vi "名称未設定 1.vi"() -> ()   [LabVIEW 2016]
panel:
  in  "FieldPoint I/Oポイント":refnum<k21>
  in  "DAQmxデバイス名":tag
  in  "クラシック従来型DAQチャンネル":tag
  in  "クラシックDAQmxデバイス名":tag
  out "波形チャート 4":dbl(graph)
  out "波形チャート 3":dbl(graph)
  out "波形チャート 2":dbl(graph)
  out "波形チャート":dbl(graph)
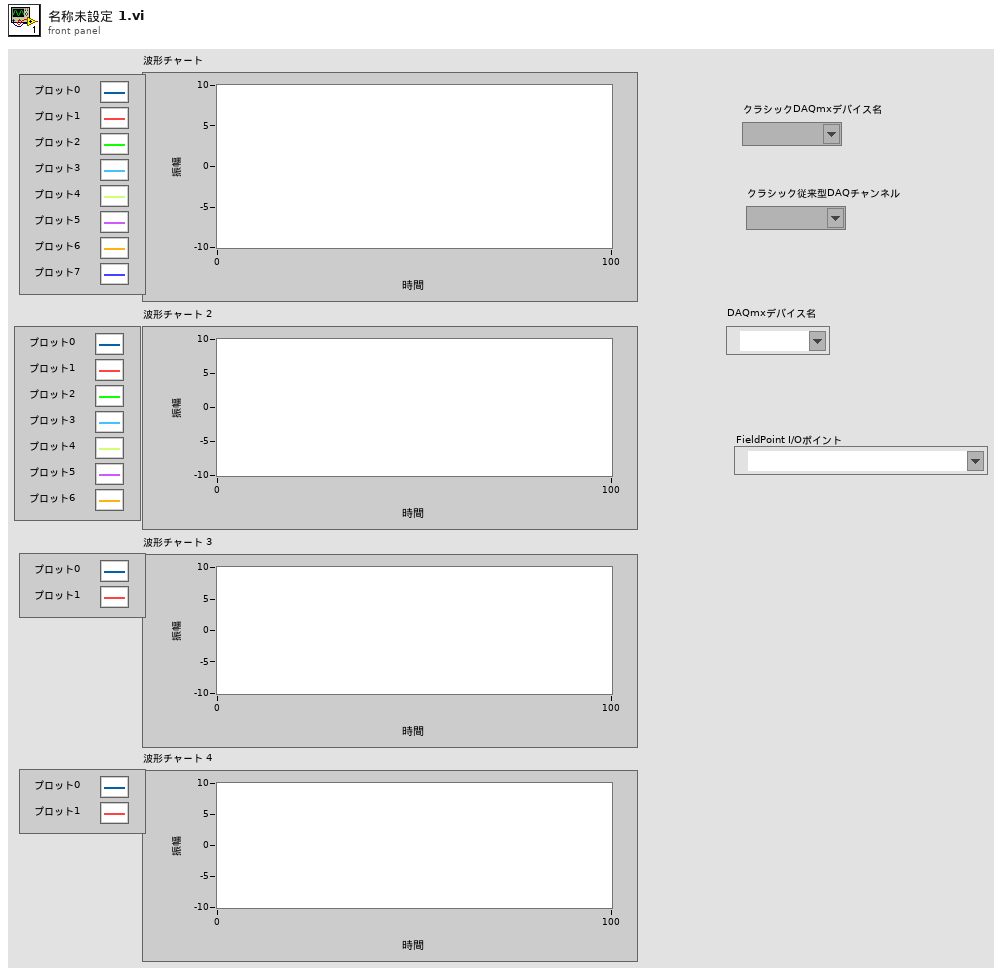
[diagram p1: front panel]
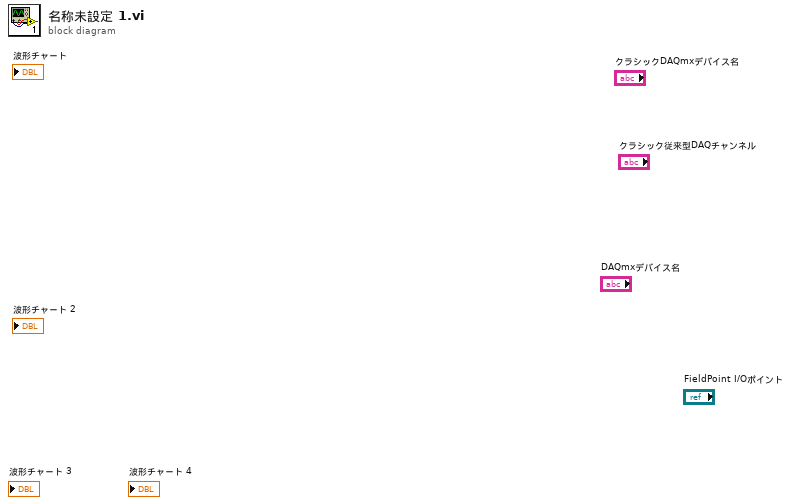
[diagram p0: block diagram]
diagram:
